vi "DD-MM-YYYY string to Timestamp.vi"(11 "String":string="25-09-2018 06:30:00") -> (3 "time stamp":timestamp)   [LabVIEW 2017]
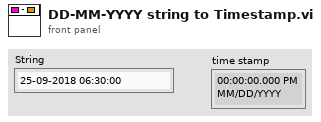
[diagram p1: front panel]
types:
  T1 = typedef "LVDateTimeRec.ctl" = cluster{"fractional second":dbl, "second":i32, "minute":i32, "hour":i32, "day of month":i32, "month":i32, "year":i32, "day of week":i32, "day of year":i32, "DST":i32}
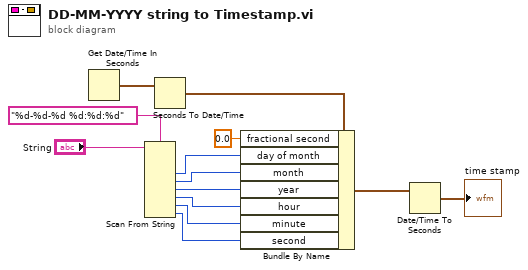
[diagram p0: block diagram]
diagram:
  n1 = Get Date/Time In Seconds() -> (seconds since 1Jan1904=w13:timestamp)
  n2 = Scan From String(format string="%d-%d-%d %d:%d:%d", input string="String") -> (output 1=w8:i32, output 2=w7:i32, output 3=w6:i32, output 4=w5:i32, output 5=w4:i32, output 6=w3:i32)  [unwired: 8 in, 3 out]
  n3 = Seconds To Date/Time(time stamp (now)=w13) -> (date time rec=w12:T1)  [unwired: 1 in]
  n4 = Bundle By Name(cluster=w12, "fractional second"=0.0, "day of month"=w8, "month"=w7, "year"=w6, "hour"=w5, "minute"=w4, "second"=w3) -> (w2:T1)
  n5 = Date/Time To Seconds(2:w2) -> (0:→"time stamp":timestamp)  [unwired: 1 in]
